vi "Sine signal generator.vi"(0 "Signal duration [sec]":i32=2, 1 "Amplitude [deg]":dbl, 2 "Frequency \n[Hz, cycles/sec]":dbl=10.0 step=1.0, 3 "Signal sampling period [ms]":i32=5 step=1, 4 "Append deceleration profile":bool=TRUE, 5 "Error In":errorcluster) -> (6 "Full sine profile":dbl[](array[numeric])=[0.0, 0.07725424859373685, 0.14694631307311828, 0.20225424859373686, 0.23776412907378838, 0.25, 0.2377641290737884, 0.20225424859373686, 0.1469463130731183, 0.07725424859373688, 3.061616997868383e-17, -0.07725424859373682, -0.14694631307311826, -0.20225424859373684, -0.23776412907378838, -0.25, -0.2377641290737884, -0.2022542485937369, -0.14694631307311834, -0.0772542485937369, -6.123233995736766e-17, 0.0772542485937368, 0.14694631307311823, 0.2022542485937368, 0.23776412907378838, 0.25, 0.2377641290737884, 0.20225424859373692, 0.14694631307311834, 0.07725424859373695, 9.184850993605148e-17, -0.07725424859373677, -0.1469463130731182, -0.2022542485937368, -0.23776412907378836, -0.25, -0.23776412907378844, -0.20225424859373692, -0.14694631307311837, -0.07725424859373697, -1.2246467991473532e-16, 0.07725424859373715, 0.14694631307311817, 0.20225424859373678, 0.23776412907378836, 0.25, 0.23776412907378844, 0.20225424859373667, 0.1469463130731184, 0.077254248593737, 1.5308084989341916e-16, -0.07725424859373713, -0.14694631307311815, -0.20225424859373703, -0.23776412907378836, -0.25, -0.23776412907378844, -0.2022542485937367, -0.14694631307311842, -0.07725424859373745, -1.8369701987210297e-16, 0.07725424859373625, 0.14694631307311812, 0.202254248593737, 0.23776412907378833, 0.25, 0.23776412907378847, 0.20225424859373672, 0.14694631307311845, 0.07725424859373664, -6.738652298493384e-16, -0.07725424859373622, -0.14694631307311812, -0.20225424859373647, -0.23776412907378833, -0.25, -0.23776412907378847, -0.20225424859373672, -0.14694631307311848, -0.07725424859373667, -2.4492935982947064e-16, 0.07725424859373704, 0.14694631307311878, 0.20225424859373697, 0.23776412907378833, 0.25, 0.23776412907378847, 0.20225424859373728, 0.1469463130731185, 0.0772542485937367, 2.755455298081545e-16, -0.07725424859373702, -0.14694631307311806, -0.20225424859373695, -0.23776412907378858, -0.25, -0.2377641290737885, -0.20225424859373728, -0.14694631307311853, -0.07725424859373757, -3.061616997868383e-16, 0.07725424859373699, 0.14694631307311876, 0.20225424859373642, 0.2377641290737883, 0.25, 0.23776412907378822, 0.20225424859373625, 0.14694631307311856, 0.07725424859373675, -5.514005499346031e-16, -0.0772542485937378, -0.146946313073118, -0.20225424859373692, -0.23776412907378855, -0.25, -0.2377641290737885, -0.20225424859373786, -0.14694631307311928, -0.07725424859373763, -3.6739403974420594e-16, 0.07725424859373693, 0.14694631307311726, 0.20225424859373636, 0.23776412907378827, 0.25, 0.23776412907378824, 0.20225424859373733, 0.1469463130731186, 0.07725424859373681, -4.901682099772354e-16, -0.07725424859373606, -0.14694631307311795, -0.2022542485937369, -0.23776412907378855, -0.25, -0.23776412907378852, -0.20225424859373684, -0.1469463130731179, -0.07725424859373599, 1.3477304596986769e-15, 0.07725424859373518, 0.1469463130731172, 0.20225424859373634, 0.23776412907378824, 0.25, 0.2377641290737888, 0.2022542485937374, 0.14694631307311865, 0.07725424859373686, 1.3474209693803826e-15, -0.07725424859373599, -0.1469463130731179, -0.20225424859373684, -0.23776412907378852, -0.25, -0.23776412907378855, -0.2022542485937369, -0.14694631307311795, -0.07725424859373606, -4.898587196589413e-16, 0.07725424859373681, 0.1469463130731186, 0.20225424859373733, 0.2377641290737888, 0.25, 0.23776412907378827, 0.20225424859373742, 0.1469463130731187, 0.07725424859373693, 1.4086533093377504e-15, -0.07725424859373593, -0.14694631307311787, -0.2022542485937368, -0.23776412907378797, -0.25, -0.23776412907378855, -0.20225424859373692, -0.146946313073118, -0.0772542485937378, -5.51091059616309e-16, 0.07725424859373675, 0.14694631307311856, 0.2022542485937373, 0.23776412907378822, 0.25, 0.2377641290737883, 0.20225424859373642, 0.1469463130731173, 0.07725424859373699, -3.064711901051325e-16, -0.07725424859373757, -0.1469463130731178, -0.20225424859373572, -0.23776412907378794, -0.25, -0.23776412907378858, -0.20225424859373695, -0.14694631307311948, -0.07725424859373786, -6.123233995736766e-16, 0.07725424859373839, 0.1469463130731185, 0.20225424859373728, 0.23776412907378874, 0.25, 0.23776412907378885, 0.2022542485937375, 0.14694631307311878, 0.07725424859373704, -2.452388501477648e-16, -0.07725424859373413, -0.1469463130731192, -0.2022542485937357, -0.23776412907378902, -0.25, -0.2377641290737886, -0.20225424859373697, -0.1469463130731181, -0.07725424859373622, 1.1028010998692062e-15, 0.07725424859373495, 0.1469463130731199, 0.2022542485937362, 0.2377641290737882, 0.25, 0.23776412907378833, 0.20225424859373647, 0.14694631307311742, 0.07725424859373879, -1.960363349590648e-15, -0.07725424859373577, -0.1469463130731177, -0.2022542485937367, -0.23776412907378736, -0.25, -0.23776412907378916, -0.20225424859373597, -0.1469463130731196, -0.07725424859373797, -7.347880794884119e-16, 0.07725424859373657, 0.1469463130731184, 0.2022542485937372, 0.2377641290737876, 0.25, 0.2377641290737889, 0.20225424859373548, 0.1469463130731189, 0.07725424859373715, -1.227741702330295e-16, -0.07725424859373739, -0.1469463130731191, -0.2022542485937377, -0.23776412907378788, -0.25, -0.23776412907378863, -0.20225424859373706, -0.1469463130731182, -0.07725424859373972, 9.803364199544708e-16, 0.07725424859373482, 0.14694631307311692, 0.2022542485937361, 0.23776412907378813, 0.25, 0.23776412907378838, 0.20225424859373864, 0.1469463130731175, 0.0772542485937389, -1.8378986696759123e-15, -0.07725424859373564, -0.14694631307311762, -0.2022542485937366, -0.2377641290737884, -0.25, -0.2377641290737881, -0.20225424859373814, -0.1469463130731168, -0.07725424859373808, 2.6954609193973537e-15, 0.07725424859373646, 0.14694631307311543, 0.20225424859373714, 0.23776412907378758, 0.25, 0.23776412907378894, 0.20225424859373764, 0.146946313073119, 0.07725424859373728, -3.0949031829417885e-19, -0.07725424859373728, -0.14694631307311612, -0.20225424859373764, -0.23776412907378783, -0.25, -0.23776412907378866, -0.20225424859373714, -0.1469463130731183, -0.07725424859373646, -2.6948419387607653e-15, 0.0772542485937381, 0.1469463130731168, 0.20225424859373814, 0.2377641290737881, 0.25, 0.2377641290737884, 0.2022542485937366, 0.14694631307311762, 0.07725424859373903, 1.837279689039324e-15, -0.07725424859373553, -0.1469463130731175, -0.20225424859373656, -0.23776412907378838, -0.25, -0.23776412907378813, -0.20225424859373822, -0.14694631307311692, -0.07725424859373821, -9.797174393178826e-16, 0.07725424859373635, 0.1469463130731182, 0.20225424859373706, 0.23776412907378863, 0.25, 0.23776412907378788, 0.2022542485937377, 0.14694631307311623, 0.07725424859373739, 1.2215518959644115e-16, -0.07725424859373715, -0.1469463130731189, -0.20225424859373756, -0.2377641290737878, -0.25, -0.23776412907378872, -0.2022542485937372, -0.1469463130731184, -0.07725424859373657, -2.8173066186755008e-15, 0.07725424859373797, 0.14694631307311673, 0.20225424859373597, 0.23776412907378808, 0.25, 0.23776412907378844, 0.2022542485937367, 0.1469463130731206, 0.07725424859373577, 1.9597443689540594e-15, -0.07725424859373879, -0.14694631307311742, -0.20225424859373647, -0.23776412907378833, -0.25, -0.2377641290737882, -0.2022542485937362, -0.1469463130731199, -0.07725424859373832, -1.102182119232618e-15, 0.07725424859373622, 0.14694631307311812, 0.2022542485937349, 0.2377641290737886, 0.25, 0.2377641290737879, 0.20225424859373778, 0.1469463130731192, 0.0772542485937375, 2.4461986951117647e-16, -0.07725424859373704, -0.1469463130731188, -0.2022542485937354, -0.23776412907378885, -0.25, -0.23776412907378766, -0.20225424859373728, -0.1469463130731185, -0.0772542485937367, 6.12942380210265e-16, 0.07725424859373448, 0.1469463130731195, 0.20225424859373592, 0.23776412907378802, 0.25, 0.23776412907378958, 0.20225424859373678, 0.14694631307312067, 0.07725424859373588, 2.0822090488687945e-15, -0.0772542485937353, -0.1469463130731173, -0.20225424859373642, -0.2377641290737883, -0.25, -0.23776412907378933, -0.20225424859373625, -0.14694631307311998, -0.07725424859373506, 0.0, 0.07351008130807599, 0.13395669874474916, 0.17953157444079718, 0.21108198137550377, 0.23096988312782168, 0.24214579028215777, 0.24750591442913938, 0.2495066821070679, 0.24996915812041515], 7 "Duration of full profile [sec]":i32=2, 8 "error out":errorcluster)   [LabVIEW 2018]
uses:
  <vilib>/Analysis/NI_AALBase.lvlib
  <vilib>/ptbypt/NI_PtbyPt.lvlib
panel:
  out "Sampled deceleration profile":dbl[](array[numeric])=[0.0, 0.07351008130807599, 0.13395669874474916, 0.17953157444079718, 0.21108198137550377, 0.23096988312782168, 0.24214579028215777, 0.24750591442913938, 0.2495066821070679, 0.24996915812041515]
  out "Deceleration profile":cluster{i32, dbl, "Chirp Pattern":dbl[]}(graph)={2, 0.005, "Chirp Pattern"=[0.0, 0.07351008130807599, 0.13395669874474916, 0.17953157444079718, 0.21108198137550377, 0.23096988312782168, 0.24214579028215777, 0.24750591442913938, 0.2495066821070679, 0.24996915812041515]}
  out "Samples in full profile":i32=410
  out "Full sine profile":cluster{"phase":dbl, dbl, dbl[]}(graph)={"phase"=0.0, 0.005, [0.0, 0.07725424859373685, 0.14694631307311828, 0.20225424859373686, 0.23776412907378838, 0.25, 0.2377641290737884, 0.20225424859373686, 0.1469463130731183, 0.07725424859373688, 3.061616997868383e-17, -0.07725424859373682, -0.14694631307311826, -0.20225424859373684, -0.23776412907378838, -0.25, -0.2377641290737884, -0.2022542485937369, -0.14694631307311834, -0.0772542485937369, -6.123233995736766e-17, 0.0772542485937368, 0.14694631307311823, 0.2022542485937368, 0.23776412907378838, 0.25, 0.2377641290737884, 0.20225424859373692, 0.14694631307311834, 0.07725424859373695, 9.184850993605148e-17, -0.07725424859373677, -0.1469463130731182, -0.2022542485937368, -0.23776412907378836, -0.25, -0.23776412907378844, -0.20225424859373692, -0.14694631307311837, -0.07725424859373697, -1.2246467991473532e-16, 0.07725424859373715, 0.14694631307311817, 0.20225424859373678, 0.23776412907378836, 0.25, 0.23776412907378844, 0.20225424859373667, 0.1469463130731184, 0.077254248593737, 1.5308084989341916e-16, -0.07725424859373713, -0.14694631307311815, -0.20225424859373703, -0.23776412907378836, -0.25, -0.23776412907378844, -0.2022542485937367, -0.14694631307311842, -0.07725424859373745, -1.8369701987210297e-16, 0.07725424859373625, 0.14694631307311812, 0.202254248593737, 0.23776412907378833, 0.25, 0.23776412907378847, 0.20225424859373672, 0.14694631307311845, 0.07725424859373664, -6.738652298493384e-16, -0.07725424859373622, -0.14694631307311812, -0.20225424859373647, -0.23776412907378833, -0.25, -0.23776412907378847, -0.20225424859373672, -0.14694631307311848, -0.07725424859373667, -2.4492935982947064e-16, 0.07725424859373704, 0.14694631307311878, 0.20225424859373697, 0.23776412907378833, 0.25, 0.23776412907378847, 0.20225424859373728, 0.1469463130731185, 0.0772542485937367, 2.755455298081545e-16, -0.07725424859373702, -0.14694631307311806, -0.20225424859373695, -0.23776412907378858, -0.25, -0.2377641290737885, -0.20225424859373728, -0.14694631307311853, -0.07725424859373757, -3.061616997868383e-16, 0.07725424859373699, 0.14694631307311876, 0.20225424859373642, 0.2377641290737883, 0.25, 0.23776412907378822, 0.20225424859373625, 0.14694631307311856, 0.07725424859373675, -5.514005499346031e-16, -0.0772542485937378, -0.146946313073118, -0.20225424859373692, -0.23776412907378855, -0.25, -0.2377641290737885, -0.20225424859373786, -0.14694631307311928, -0.07725424859373763, -3.6739403974420594e-16, 0.07725424859373693, 0.14694631307311726, 0.20225424859373636, 0.23776412907378827, 0.25, 0.23776412907378824, 0.20225424859373733, 0.1469463130731186, 0.07725424859373681, -4.901682099772354e-16, -0.07725424859373606, -0.14694631307311795, -0.2022542485937369, -0.23776412907378855, -0.25, -0.23776412907378852, -0.20225424859373684, -0.1469463130731179, -0.07725424859373599, 1.3477304596986769e-15, 0.07725424859373518, 0.1469463130731172, 0.20225424859373634, 0.23776412907378824, 0.25, 0.2377641290737888, 0.2022542485937374, 0.14694631307311865, 0.07725424859373686, 1.3474209693803826e-15, -0.07725424859373599, -0.1469463130731179, -0.20225424859373684, -0.23776412907378852, -0.25, -0.23776412907378855, -0.2022542485937369, -0.14694631307311795, -0.07725424859373606, -4.898587196589413e-16, 0.07725424859373681, 0.1469463130731186, 0.20225424859373733, 0.2377641290737888, 0.25, 0.23776412907378827, 0.20225424859373742, 0.1469463130731187, 0.07725424859373693, 1.4086533093377504e-15, -0.07725424859373593, -0.14694631307311787, -0.2022542485937368, -0.23776412907378797, -0.25, -0.23776412907378855, -0.20225424859373692, -0.146946313073118, -0.0772542485937378, -5.51091059616309e-16, 0.07725424859373675, 0.14694631307311856, 0.2022542485937373, 0.23776412907378822, 0.25, 0.2377641290737883, 0.20225424859373642, 0.1469463130731173, 0.07725424859373699, -3.064711901051325e-16, -0.07725424859373757, -0.1469463130731178, -0.20225424859373572, -0.23776412907378794, -0.25, -0.23776412907378858, -0.20225424859373695, -0.14694631307311948, -0.07725424859373786, -6.123233995736766e-16, 0.07725424859373839, 0.1469463130731185, 0.20225424859373728, 0.23776412907378874, 0.25, 0.23776412907378885, 0.2022542485937375, 0.14694631307311878, 0.07725424859373704, -2.452388501477648e-16, -0.07725424859373413, -0.1469463130731192, -0.2022542485937357, -0.23776412907378902, -0.25, -0.2377641290737886, -0.20225424859373697, -0.1469463130731181, -0.07725424859373622, 1.1028010998692062e-15, 0.07725424859373495, 0.1469463130731199, 0.2022542485937362, 0.2377641290737882, 0.25, 0.23776412907378833, 0.20225424859373647, 0.14694631307311742, 0.07725424859373879, -1.960363349590648e-15, -0.07725424859373577, -0.1469463130731177, -0.2022542485937367, -0.23776412907378736, -0.25, -0.23776412907378916, -0.20225424859373597, -0.1469463130731196, -0.07725424859373797, -7.347880794884119e-16, 0.07725424859373657, 0.1469463130731184, 0.2022542485937372, 0.2377641290737876, 0.25, 0.2377641290737889, 0.20225424859373548, 0.1469463130731189, 0.07725424859373715, -1.227741702330295e-16, -0.07725424859373739, -0.1469463130731191, -0.2022542485937377, -0.23776412907378788, -0.25, -0.23776412907378863, -0.20225424859373706, -0.1469463130731182, -0.07725424859373972, 9.803364199544708e-16, 0.07725424859373482, 0.14694631307311692, 0.2022542485937361, 0.23776412907378813, 0.25, 0.23776412907378838, 0.20225424859373864, 0.1469463130731175, 0.0772542485937389, -1.8378986696759123e-15, -0.07725424859373564, -0.14694631307311762, -0.2022542485937366, -0.2377641290737884, -0.25, -0.2377641290737881, -0.20225424859373814, -0.1469463130731168, -0.07725424859373808, 2.6954609193973537e-15, 0.07725424859373646, 0.14694631307311543, 0.20225424859373714, 0.23776412907378758, 0.25, 0.23776412907378894, 0.20225424859373764, 0.146946313073119, 0.07725424859373728, -3.0949031829417885e-19, -0.07725424859373728, -0.14694631307311612, -0.20225424859373764, -0.23776412907378783, -0.25, -0.23776412907378866, -0.20225424859373714, -0.1469463130731183, -0.07725424859373646, -2.6948419387607653e-15, 0.0772542485937381, 0.1469463130731168, 0.20225424859373814, 0.2377641290737881, 0.25, 0.2377641290737884, 0.2022542485937366, 0.14694631307311762, 0.07725424859373903, 1.837279689039324e-15, -0.07725424859373553, -0.1469463130731175, -0.20225424859373656, -0.23776412907378838, -0.25, -0.23776412907378813, -0.20225424859373822, -0.14694631307311692, -0.07725424859373821, -9.797174393178826e-16, 0.07725424859373635, 0.1469463130731182, 0.20225424859373706, 0.23776412907378863, 0.25, 0.23776412907378788, 0.2022542485937377, 0.14694631307311623, 0.07725424859373739, 1.2215518959644115e-16, -0.07725424859373715, -0.1469463130731189, -0.20225424859373756, -0.2377641290737878, -0.25, -0.23776412907378872, -0.2022542485937372, -0.1469463130731184, -0.07725424859373657, -2.8173066186755008e-15, 0.07725424859373797, 0.14694631307311673, 0.20225424859373597, 0.23776412907378808, 0.25, 0.23776412907378844, 0.2022542485937367, 0.1469463130731206, 0.07725424859373577, 1.9597443689540594e-15, -0.07725424859373879, -0.14694631307311742, -0.20225424859373647, -0.23776412907378833, -0.25, -0.2377641290737882, -0.2022542485937362, -0.1469463130731199, -0.07725424859373832, -1.102182119232618e-15, 0.07725424859373622, 0.14694631307311812, 0.2022542485937349, 0.2377641290737886, 0.25, 0.2377641290737879, 0.20225424859373778, 0.1469463130731192, 0.0772542485937375, 2.4461986951117647e-16, -0.07725424859373704, -0.1469463130731188, -0.2022542485937354, -0.23776412907378885, -0.25, -0.23776412907378766, -0.20225424859373728, -0.1469463130731185, -0.0772542485937367, 6.12942380210265e-16, 0.07725424859373448, 0.1469463130731195, 0.20225424859373592, 0.23776412907378802, 0.25, 0.23776412907378958, 0.20225424859373678, 0.14694631307312067, 0.07725424859373588, 2.0822090488687945e-15, -0.0772542485937353, -0.1469463130731173, -0.20225424859373642, -0.2377641290737883, -0.25, -0.23776412907378933, -0.20225424859373625, -0.14694631307311998, -0.07725424859373506, 0.0, 0.07351008130807599, 0.13395669874474916, 0.17953157444079718, 0.21108198137550377, 0.23096988312782168, 0.24214579028215777, 0.24750591442913938, 0.2495066821070679, 0.24996915812041515]}
  # "INPUTS"
  # "OUTPUTS"
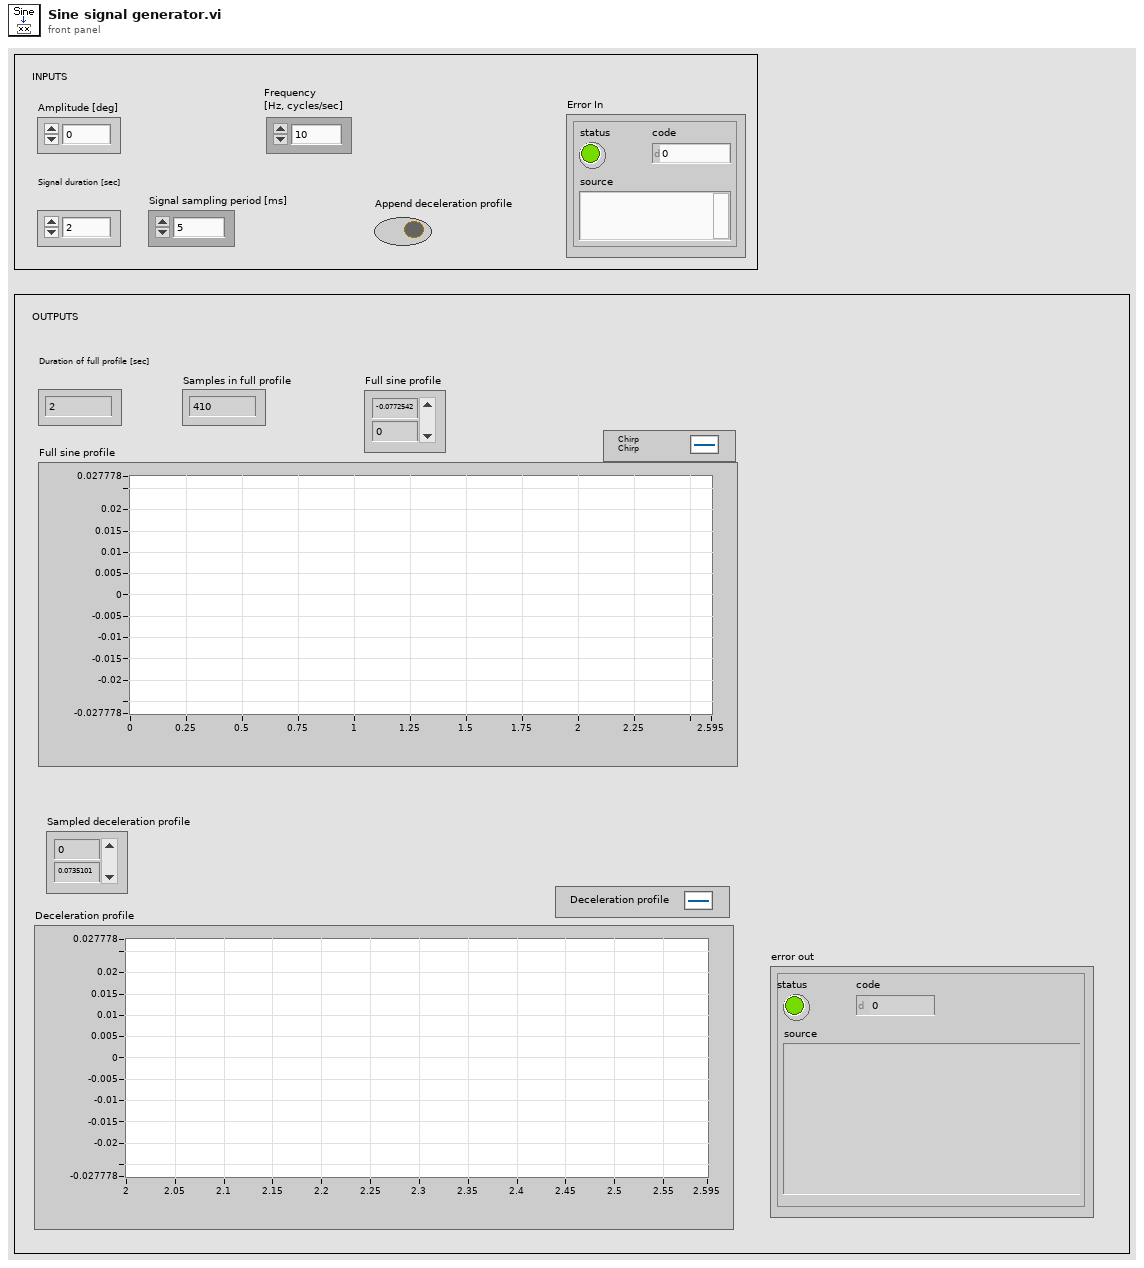
[diagram p1: front panel]
types:
  T1 = cluster{"Signal duration [sec]":i32, dbl, "Chirp Pattern":dbl[]}
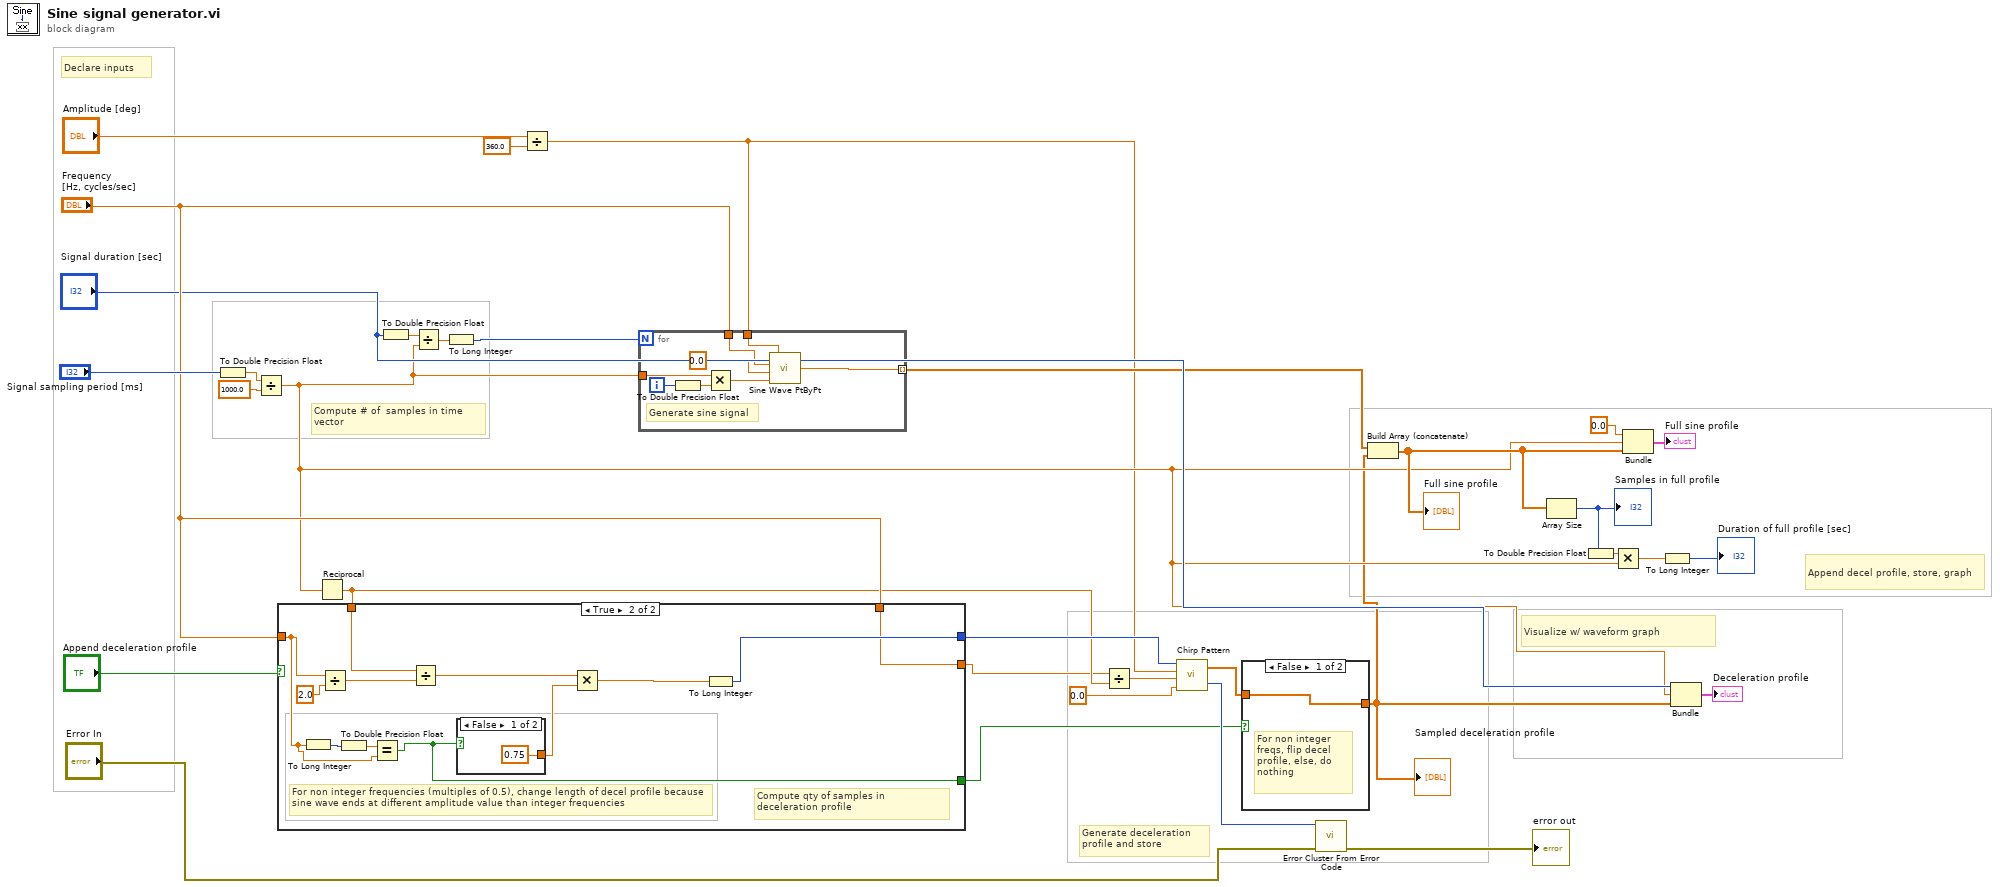
[diagram p0: block diagram]
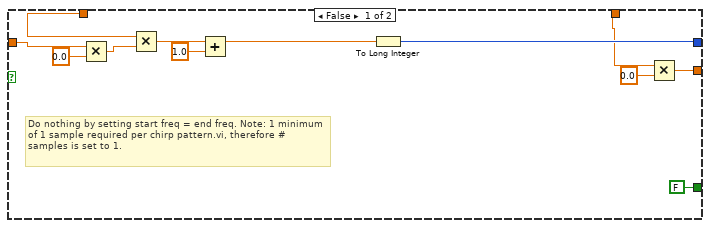
[diagram p3: hidden frame]
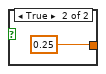
[diagram p4: hidden frame]
diagram:
  # "For non integer freqs, flip decel profile, else, do nothing"
  # "Compute # of  samples in time vector"
  # "Generate deceleration profile and store"
  # "Visualize w/ waveform graph"
  # "Append decel profile, store, graph"
  # "Declare inputs"
  n1 = To Double Precision Float(number="Signal sampling period [ms]") -> (double precision float=w14:dbl)
  n2 = Divide(x=w14, y=1000.0) -> (x/y=w6:dbl)
  n3 = Reciprocal(x=w6) -> (1/x=w9:dbl)
  n4 = case shown="True" "Append deceleration profile" {
    tunnel: "Frequency \n[Hz, cycles/sec]" -> [w45 w48]
    tunnel: w9 -> [w43 w53]
    tunnel: [w40 w52] -> w24
    tunnel: "Frequency \n[Hz, cycles/sec]" -> [w36 w51]
    tunnel: [w35 w51] -> w7
    tunnel: [FALSE w47] -> w3
    frame False {
      # "Do nothing by setting start freq = end freq. Note: 1 minimum of 1 sample required per chirp pattern.vi, therefore # samples is set to 1."
      n5 = Multiply(x=w45, y=0.0) -> (x*y=w42:dbl)
      n6 = Multiply(x=w43, y=w42) -> (x*y=w41:dbl)
      n7 = Add(x=w41, y=1.0) -> (x+y=w39:dbl)
      n8 = To Long Integer(number=w39) -> (32bit integer=w40:i32)
      n9 = Multiply(x=w36, y=0.0) -> (x*y=w35:dbl)
    }
    frame True {
      # "For non integer frequencies (multiples of 0.5), change length of decel profile because sine wave ends at different amplitude value than integer frequencies"
      # "Compute qty of samples in deceleration profile"
      n10 = To Long Integer(number=w48) -> (32bit integer=w50:i32)
      n11 = Divide(x=w48, y=2.0) -> (x/y=w56:dbl)
      n12 = To Double Precision Float(number=w50) -> (double precision float=w49:dbl)
      n13 = Equal?(x=w49, y=w48) -> (x = y?=w47:bool)
      n14 = Divide(x=w53, y=w56) -> (x/y=w55:dbl)
      n15 = case shown="False" w47 {
        tunnel: [0.75 ("y") 0.25 ("y")] -> w46
        frame False {
        }
        frame True {
        }
      }
      n16 = Multiply(x=w55, y=w46) -> (x*y=w54:dbl)
      n17 = To Long Integer(number=w54) -> (32bit integer=w52:i32)
    }
  }
  n18 = To Double Precision Float(number="Signal duration [sec]") -> (double precision float=w18:dbl)
  n19 = Divide(x=w18, y=w6) -> (x/y=w15:dbl)
  n20 = To Long Integer(number=w15) -> (32bit integer=w17:i32)
  n21 = Divide(x="Amplitude [deg]", y=360.0) -> (x/y=w5:dbl)
  n22 = for {
    N: w17 -> [_]
    tunnel: w6 -> [w65]
    tunnel: "Frequency \n[Hz, cycles/sec]" -> [w63]
    tunnel: w5 -> [w62]
    tunnel: [w60] -> w10 mode=indexing
    i -> [w67]
    # "Generate sine signal"
    n23 = To Double Precision Float(number=w67) -> (double precision float=w66:dbl)
    n24 = Multiply(x=w65, y=w66) -> (x*y=w61:dbl)
    n25 = call <vilib>:"Sine Wave PtByPt.vi"("time"=w61, "phase"=0.0, "frequency"=w63, "amplitude"=w62) -> ("sine wave"=w60:dbl)
  }
  n26 = Divide(x=w7, y=w9) -> (x/y=w8:dbl)
  n27 = call <vilib>:"Chirp Pattern.vi"("f2"=0.0, "f1"=w8, "amplitude"=w5, "samples"=w24) -> ("error"=w25:i32, "Chirp Pattern"=w2:dbl[])
  n28 = case shown="False" w3 {
    tunnel: w2 -> [w68 w69]
    tunnel: [w68 w69] -> w1
    frame False {
    }
    frame True {
    }
  }
  "Sampled deceleration profile" <- w1
  n29 = call <vilib>:"Error Cluster From Error Code.vi"("error in (no error)"="Error In", "error code (0)"=w25) -> ("error out"=→"error out":errorcluster)  [unwired: 7 in]
  n30 = Build Array (concatenate)(w10, w1) -> (w29:dbl[])
  "Full sine profile" <- w29
  n31 = Array Size(array=w29) -> (size(s)=w28:i32)
  "Samples in full profile" <- w28
  n32 = To Double Precision Float(number=w28) -> (double precision float=w19:dbl)
  n33 = Multiply(x=w19, y=w6) -> (x*y=w21:dbl)
  n34 = Bundle("phase"=0.0, w6, w29) -> (→"Full sine profile":cluster{"phase":dbl, dbl, dbl[]})  [unwired: 1 in]
  n35 = To Long Integer(number=w21) -> (32bit integer=→"Duration of full profile [sec]":i32)
  n36 = Bundle("Signal duration [sec]"="Signal duration [sec]", w6, "Chirp Pattern"=w1) -> (→"Deceleration profile":T1)  [unwired: 1 in]
